vi "Create FIFO Instance.vi"(6 "timeout (ms)":i32=5000, 8 "error in":errorcluster, 10 "New FIFO Instance":T1, 11 "gRPC ID":T2) -> (0 "error out":errorcluster, 2 "publisher_instance_name":string, 3 "gRPC ID out":T2)   [LabVIEW 2021, in "CIFCoreWrapper.lvlib"]
uses:
  CIFCoreWrapper.lvlib
  CIFCoreChannel_client/CIFCoreChannel_client.lvlib
  <vilib>/gRPC/LabVIEW gRPC Library/Shared/grpcId.ctl
  <vilib>/gRPC/LabVIEW gRPC Library/grpc-lvsupport-release.lvlib
  CIFCoreChannel_client/RPC Messages/cif_channelcore_FIFOInstance.ctl
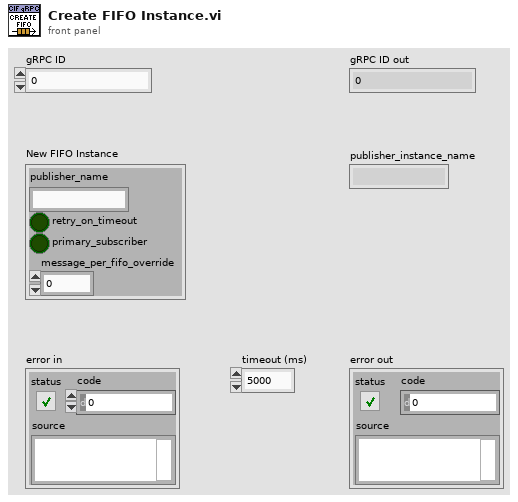
[diagram p1: front panel]
types:
  T1 = typedef "CIFCoreChannel_client.lvlib/cif_channelcore_FIFOInstance.ctl" = cluster{"publisher_name":string, "retry_on_timeout":bool, "primary_subscriber":bool, "message_per_fifo_override":u32}
  T2 = typedef "grpc-lvsupport-release.lvlib/grpcId.ctl" = u64
  T3 = typedef "CIFCoreChannel_client.lvlib/cif_channelcore_FIFOReference.ctl" = cluster{"publisher_instance_name":string, "status":T4}
  T4 = typedef "CIFCoreChannel_client.lvlib/cif_common_Status.ctl" = cluster{"code":i32, "message":string}
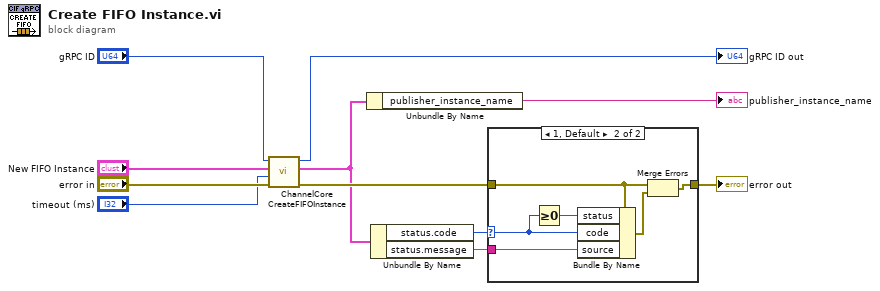
[diagram p0: block diagram]
diagram:
  n1 = call "ChannelCore CreateFIFOInstance.vi"("error in"="error in", "timeout (ms)"="timeout (ms)", "Request Data"="New FIFO Instance", "gRPC ID"="gRPC ID") -> ("error out"=w6:errorcluster, "Response Data"=w2:T3, "gRPC ID out"=→"gRPC ID out":T2)  [unwired: 5 in]
  n2 = Unbundle By Name(w2) -> ("publisher_instance_name"=→"publisher_instance_name":string)
  n3 = Unbundle By Name(w2) -> ("status.code"=w4:i32, "status.message"=w7:string)
  n4 = case shown="1, Default" w4 {
    selector: w4 -> [_ w13]
    tunnel: w7 -> [_ w17]
    tunnel: w6 -> [w12 w16]
    tunnel: [w12 w14] -> w5
    frame 0 {
    }
    frame 1, Default {
      n5 = Greater Or Equal To 0?(x=w13) -> (x >= 0?=w18:bool)
      n6 = Bundle By Name(cluster=w16, "status"=w18, "code"=w13, "source"=w17) -> (w15:errorcluster)
      n7 = Merge Errors(w16, w15) -> (w14:errorcluster)
    }
  }
  "error out" <- w5
